vi "Rad_a_Grad.vi"(1 "Radianes":dbl) -> (0 "Grados":dbl)   [LabVIEW 2020]
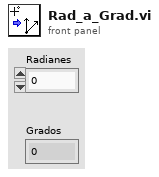
[diagram p1: front panel]
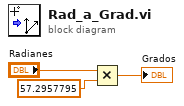
[diagram p0: block diagram]
diagram:
  n1 = Multiply(x="Radianes", y=57.2957795) -> (x*y=→"Grados":dbl)
